vi "getSheet.vi"(8 "error in (no error)":errorcluster, 10 "Sheet Index":i32, 11 "MS-Excel in":refnum<class "MS-Excel.lvclass">) -> (0 "error out":errorcluster, 2 "Sheet Ref":refnum<k24>, 3 "MS-Excel out":refnum<class "MS-Excel.lvclass">)   [LabVIEW 2017, in "LabVIEW NPOI.lvlib" / "MS-Excel.lvclass"]
uses:
  MS-Excel.lvclass
  C:/Users/Neo/Desktop/Dev_Tools_BR/LabVIEW_NPOI/lib/NPOI 2.1.1/NPOI.dll
  lib/NPOI 2.1.1/NPOI.dll
  MS-Excel.lvclass/MS-Excel.ctl
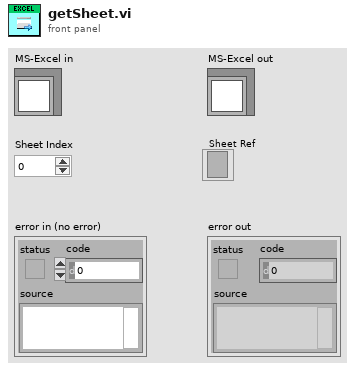
[diagram p1: front panel]
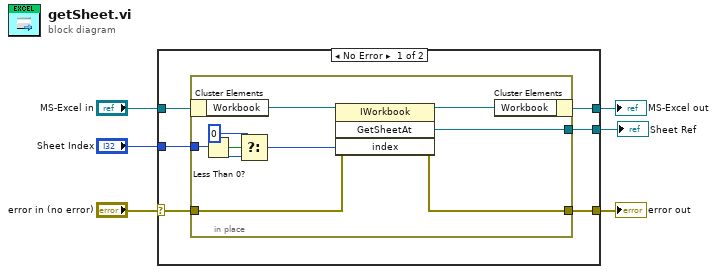
[diagram p0: block diagram]
diagram:
  n1 = case shown="No Error" "error in (no error)" {
    selector: "error in (no error)" -> [w9 w22]
    tunnel: [w8 w22] -> w6
    tunnel: [w12 w23] -> w4
    tunnel: "MS-Excel in" -> [w11 w23]
    tunnel: "Sheet Index" -> [w10 _]
    tunnel: [w7 _] -> w1
    frame No Error {
      n2 = in-place {
        in-place-border: w10 -> [w15]
        in-place-border: w9 -> [w19]
        in-place-border: [w18] -> w8
        in-place-border: [w17] -> w7
        n3 = in-place-cluster #1(w11) -> ("Workbook"=w21:refnum<k24>)
        n4 = Less Than 0?(x=w15) -> (x < 0?=w16:bool)
        n5 = Select(t=0, s=w16, f=w15) -> (s? t:f=w13:i32)
        n6 = invoke class="IWorkbook" method="GetSheetAt"(reference=w21, error in=w19, "index"=w13) -> (reference out=w20:refnum<k24>, error out=w18:errorcluster, "GetSheetAt"=w17:refnum<k24>)  [unwired: 1 in, 1 out]
        n7 = in-place-cluster #1("Workbook"=w20) -> (w12:refnum<class "MS-Excel.lvclass">)
      }
    }
    frame Error {
    }
  }
  "error out" <- w6
  "MS-Excel out" <- w4
  "Sheet Ref" <- w1
